vi "Create Accuracy Results Summary Table.vi"(8 "error in (no error)":errorcluster, 11 "Accuracy Results":T1[](array[typedef]) {"Accuracy Percent FS" format="%#_3g"}) -> (0 "error out":errorcluster, 3 "Accuracy Table":string[][](array[string]))   [LabVIEW 2026, in "Analysis.lvlib"]
uses:
  Analysis.lvlib
  Accuracy Result.ctl
panel:
  out "sorted array":dbl[](array[numeric])
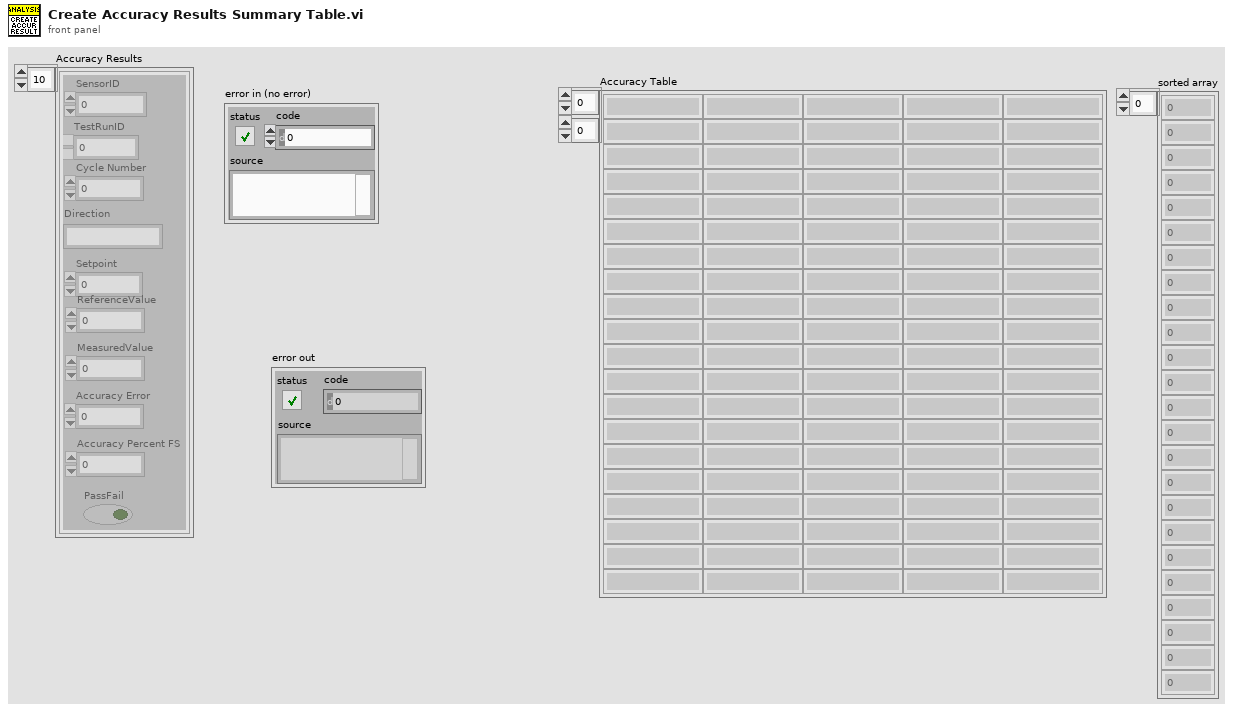
[diagram p1: front panel]
types:
  T1 = typedef "Analysis.lvlib/Accuracy Result.ctl" = cluster{"Setpoint":dbl, "Cycle Number":i32, "SensorID":i32, "TestRunID":i32, "ReferenceValue":dbl, "MeasuredValue":dbl, "Accuracy Percent FS":dbl, "PassFail":bool, "Accuracy Error":dbl, "Direction":string}
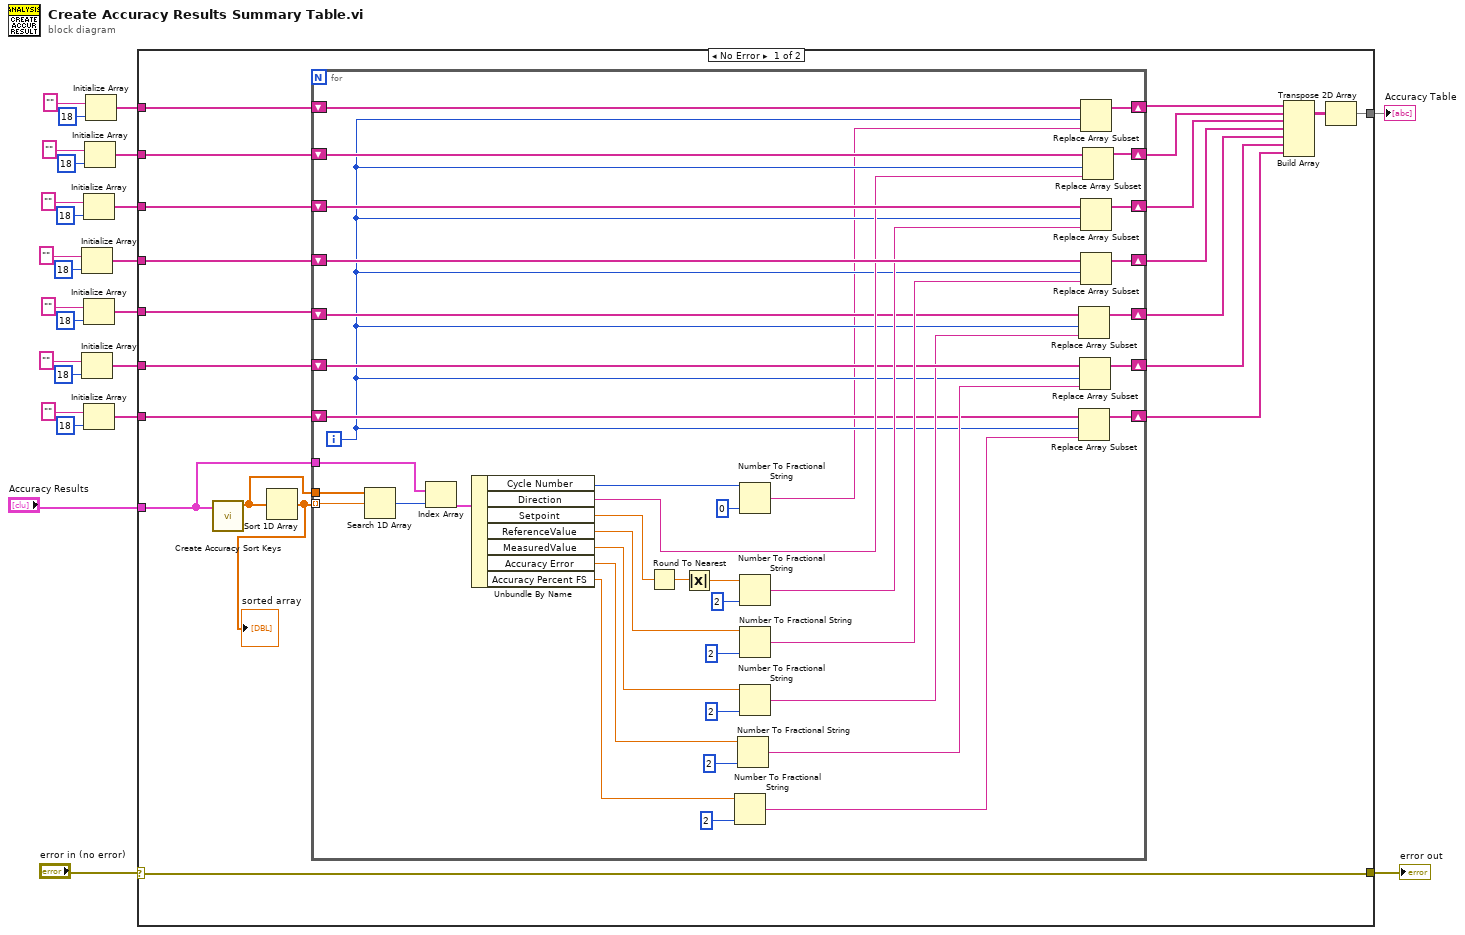
[diagram p0: block diagram]
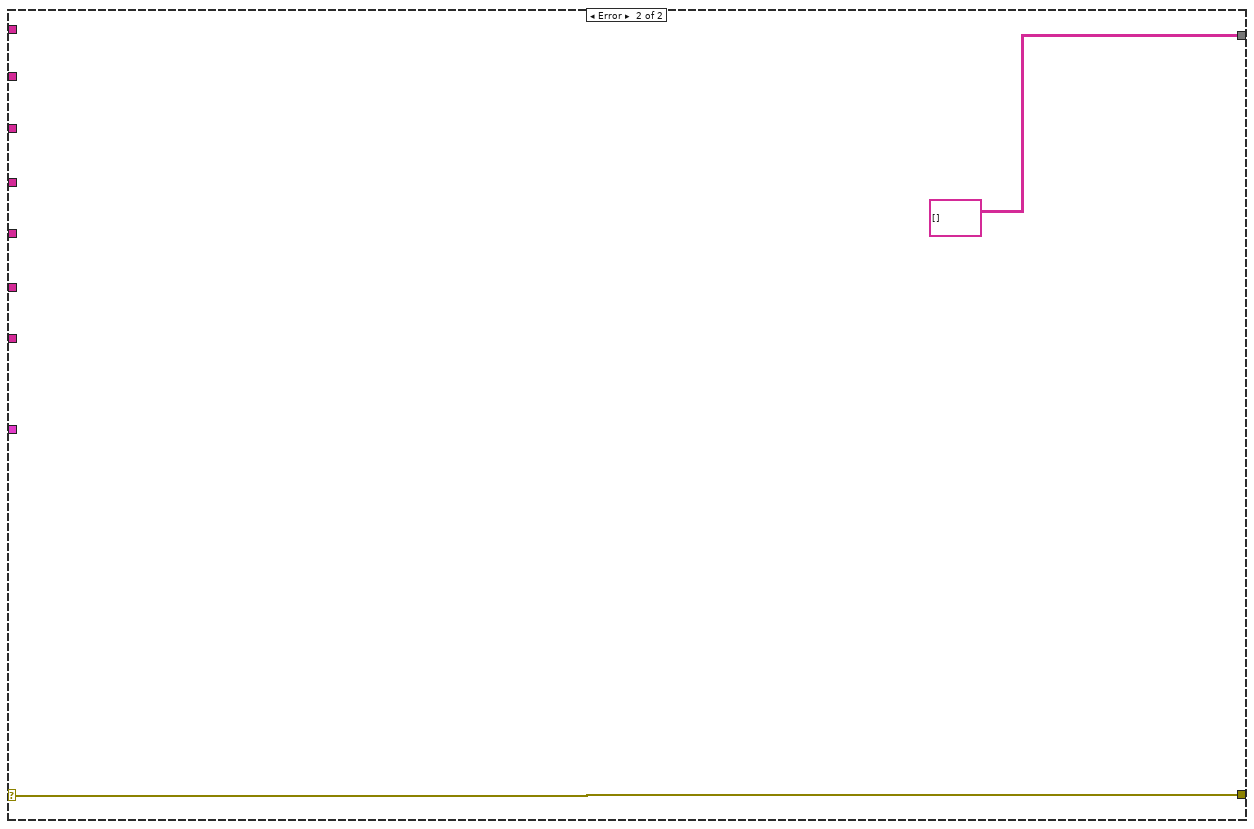
[diagram p2: hidden frame]
diagram:
  n1 = Initialize Array("" ("element"), 18 ("dimension size")) -> (w11:string[])
  n2 = Initialize Array("" ("element"), 18 ("dimension size")) -> (w5:string[])
  n3 = Initialize Array("" ("element"), 18 ("dimension size")) -> (w14:string[])
  n4 = Initialize Array("" ("element"), 18 ("dimension size")) -> (w6:string[])
  n5 = Initialize Array("" ("element"), 18 ("dimension size")) -> (w2:string[])
  n6 = Initialize Array("" ("element"), 18 ("dimension size")) -> (w20:string[])
  n7 = Initialize Array("" ("element"), 18 ("dimension size")) -> (w23:string[])
  n8 = case shown="No Error" "error in (no error)" {
    selector: "error in (no error)" -> [w39 w88]
    tunnel: w23 -> [w45 _]
    tunnel: w20 -> [w44 _]
    tunnel: "Accuracy Results" -> [w26 _]
    tunnel: [w40 string[][] []] -> w19
    tunnel: [w39 w88] -> w17
    tunnel: w14 -> [w38 _]
    tunnel: w11 -> [w36 _]
    tunnel: w6 -> [w32 _]
    tunnel: w5 -> [w30 _]
    tunnel: w2 -> [w29 _]
    frame No Error {
      n9 = call "Create Accuracy Sort Keys.vi"("Accuracy Results"=w26) -> ("Sort Keys"=w33:dbl[])  [unwired: 9 in, 1 out]
      n10 = Sort 1D Array(array=w33) -> (sorted array=w34:dbl[])
      "sorted array" <- w34
      n11 = for {
        shift-right: [w85] -> w43
        shift-left: w45 -> [w86]
        shift-right: [w83] -> w42
        shift-left: w44 -> [w84]
        shift-right: [w81] -> w37
        shift-left: w38 -> [w82]
        shift-right: [w79] -> w35
        shift-left: w36 -> [w80]
        tunnel: w34 -> [w76] mode=indexing
        tunnel: w33 -> [w75]
        tunnel: w26 -> [w73]
        shift-right: [w55] -> w31
        shift-left: w32 -> [w56]
        shift-right: [w53] -> w28
        shift-left: w30 -> [w54]
        shift-right: [w49] -> w27
        shift-left: w29 -> [w48]
        i -> [w47]
        n12 = Search 1D Array(1D array=w75, element=w76) -> (index of element=w74:i32)  [unwired: 1 in]
        n13 = Index Array(array=w73, index=w74) -> (element=w69:T1)
        n14 = Unbundle By Name(w69) -> ("Cycle Number"=w68:i32, "Direction"=w67:string, "Setpoint"=w66:dbl, "ReferenceValue"=w63:dbl, "MeasuredValue"=w61:dbl, "Accuracy Error"=w58:dbl, "Accuracy Percent FS"=w57:dbl)
        n15 = Round To Nearest(number=w66) -> (nearest integer value=w65:dbl)
        n16 = Absolute Value(x=w65) -> (abs(x)=w64:dbl)
        n17 = Number To Fractional String(number=w57, precision (6)=i16 2) -> (F-format string=w50:string)  [unwired: 2 in]
        n18 = Number To Fractional String(number=w58, precision (6)=i16 2) -> (F-format string=w51:string)  [unwired: 2 in]
        n19 = Number To Fractional String(number=w68, precision (6)=i16 0) -> (F-format string=w46:string)  [unwired: 2 in]
        n20 = Number To Fractional String(number=w64, precision (6)=i16 2) -> (F-format string=w78:string)  [unwired: 2 in]
        n21 = Number To Fractional String(number=w63, precision (6)=i16 2) -> (F-format string=w77:string)  [unwired: 2 in]
        n22 = Number To Fractional String(number=w61, precision (6)=i16 2) -> (F-format string=w52:string)  [unwired: 2 in]
        n23 = Replace Array Subset(array=w56, new element=w52, index=w47) -> (w55:string[])
        n24 = Replace Array Subset(array=w48, new element=w50, index=w47) -> (w49:string[])
        n25 = Replace Array Subset(array=w54, new element=w51, index=w47) -> (w53:string[])
        n26 = Replace Array Subset(array=w86, new element=w46, index=w47) -> (w85:string[])
        n27 = Replace Array Subset(array=w82, new element=w78, index=w47) -> (w81:string[])
        n28 = Replace Array Subset(array=w80, new element=w77, index=w47) -> (w79:string[])
        n29 = Replace Array Subset(array=w84, new element=w67, index=w47) -> (w83:string[])
      }
      n30 = Build Array(w43, w42, w37, w35, w31, w28, w27) -> (w41:string[][])
      n31 = Transpose 2D Array(2D array=w41) -> (transposed array=w40:string[][])
    }
    frame Error {
    }
  }
  "Accuracy Table" <- w19
  "error out" <- w17
